vi "LaudaDAQ.vi"(7 "device name":tag="cDAQ9188XT-1C3BF19Mod1") -> (0 "error out":errorcluster, 1 "Tj out":dbl, 2 "data":dynamicdata(waveform), 3 "Sensor OK":bool, 4 "Tj out":dbl, 5 "T external 2":dbl)   [LabVIEW 2016]
panel:
  out "Numeric":dbl
  # "cDAQ9188XT-1C3BF2FMod1"
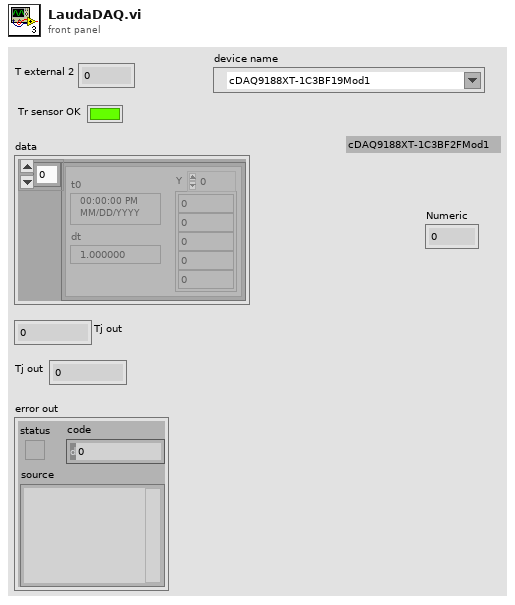
[diagram p1: front panel]
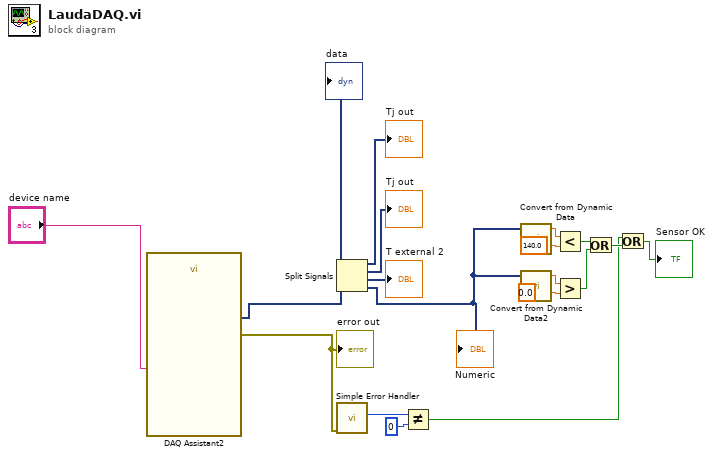
[diagram p0: block diagram]
diagram:
  n1 = call "DAQ Assistant2"("device name"="device name") -> ("data"=w13:dynamicdata, "error out"=w12:errorcluster)  [unwired: 16 in, 1 out]
  "error out" <- w12
  "data" <- w13
  n2 = Split Signals(w13) -> (→"Tj out":dynamicdata, →"Tj out":dynamicdata, →"T external 2":dynamicdata, w5:dynamicdata)  [unwired: 4 in]
  "Numeric" <- w5
  n3 = call <vilib>:"Simple Error Handler.vi"("error in (no error)"=w12) -> ("code out"=w14:i32)  [unwired: 4 in, 4 out]
  n4 = Not Equal?(x=w14, y=0) -> (x != y?=w2:bool)
  n5 = call "Convert from Dynamic Data"("Dynamic Data Type"=w5) -> ("Scalar"=w6:dbl)  [unwired: 3 in]
  n6 = call "Convert from Dynamic Data2"("Dynamic Data Type"=w5) -> ("Scalar"=w4:dbl)  [unwired: 3 in]
  n7 = Less?(x=w6, y=140.0) -> (x < y?=w8:bool)
  n8 = Greater?(x=w4, y=0.0) -> (0:w7:bool)
  n9 = Or(x=w8, y=w7) -> (x .or. y?=w3:bool)
  n10 = Or(x=w2, y=w3) -> (x .or. y?=→"Sensor OK":bool)
